vi "DataPath.vi"() -> (2 "DataDirectory":path)   [LabVIEW 2017, in "Server.lvlib"]
doc: "This VI generates a Path for the Data-Folder that contains all necessary Data-Files.\nThe Data-Folder might change from the default Application Directory to some other place (e.g. Appdata). That can easily be changed within this VI."
uses:
  Server.lvlib
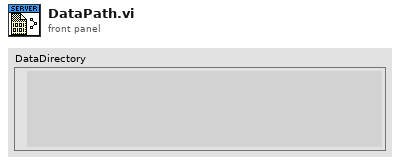
[diagram p1: front panel]
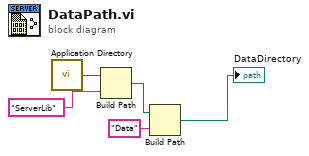
[diagram p0: block diagram]
diagram:
  n1 = call <vilib>:"Application Directory.vi"() -> ("Application Directory"=w5:path)
  n2 = Build Path(base path=w5, name or relative path="ServerLib") -> (appended path=w3:path)
  n3 = Build Path(base path=w3, name or relative path="Data") -> (appended path=→"DataDirectory":path)
